vi "Create Function String (User Defined).vi"(8 "error in (no error)":errorcluster, 10 "Function (1: F1)":i32(ring)=1 items=["F1"=1, "F2"=2, "F3"=3, "F4"=4, "F5"=5, "F6"=6, "F7"=7, "F8"=8, "F9"=9, "F10"=10, "F11"=11, "F12"=12, "F13"=13, "F14"=14, "F15"=15, "F16"=16, "F17"=17, "F18"=18, "F19"=19, "F20"=20], 11 "VISA resource name":refnum<visa-resource-name>) -> (0 "error out":errorcluster, 2 "Function String":string, 3 "VISA resource name out":refnum<visa-resource-name>)   [LabVIEW 2021, in "Yokogawa WT1800 Series.lvlib"]
doc: "Create a user define function string"
uses:
  <instrlib>/Yokogawa WT1800 Series/Yokogawa WT1800 Series.lvlib
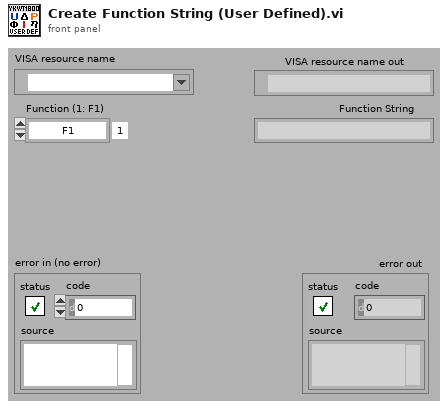
[diagram p1: front panel]
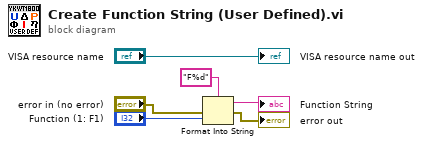
[diagram p0: block diagram]
diagram:
  n1 = Format Into String(format string="F%d" ("形式文字列"), error in="error in (no error)", "Function (1: F1)") -> (resulting string=→"Function String":string, error out=→"error out":errorcluster)  [unwired: 1 in]
  "VISA resource name out" <- "VISA resource name"
